vi "AngleStats_AngleMean_BiFunc.vi"(9 "B":T1, 10 "A":T1, 11 "ExtraPassedData":variant) -> (0 "Error":bool, 3 "Result":T1)   [LabVIEW 2019, in "Trajectory_Library.lvlib"]
doc: "Creates a new LINEAR SYSTEM data cluster with the specified values. \n\n\nInputs: \n - XXX -- XXX.\n\nOutputs:\n - XXX -- XXX."
uses:
  Trajectory_Library.lvlib
  <vilib>/Analysis/Matrix/Datatypes/RealMatrix.ctl
  <vilib>/Analysis/Matrix/NI_Matrix.lvlib
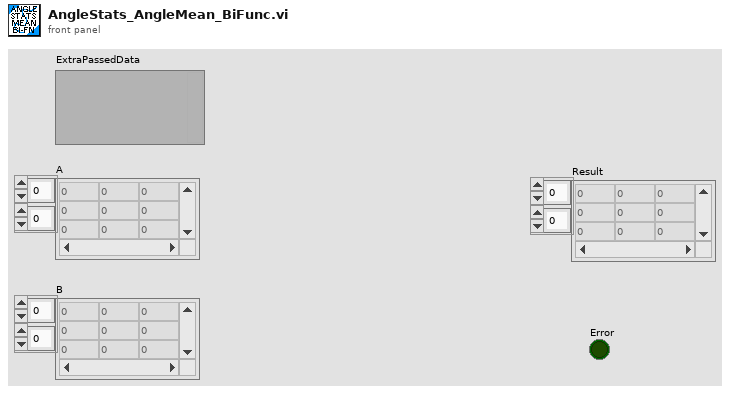
[diagram p1: front panel]
types:
  T1 = typedef "NI_Matrix.lvlib/RealMatrix.ctl" = dbl[][]
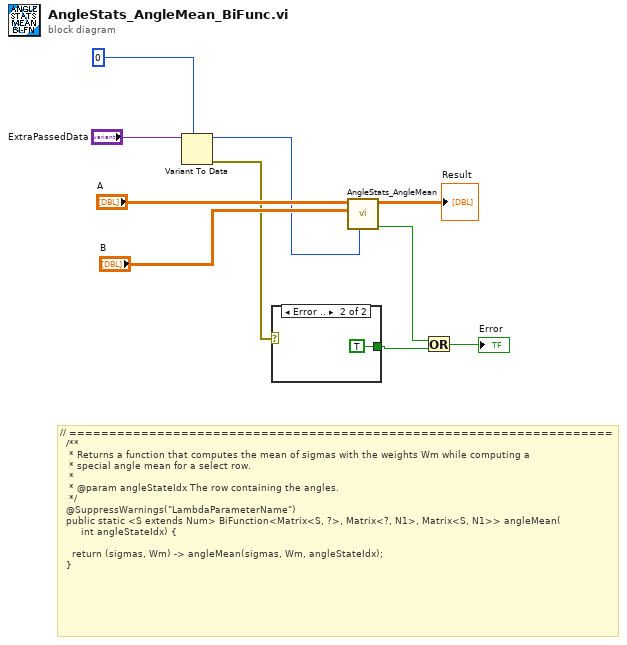
[diagram p0: block diagram]
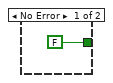
[diagram p2: hidden frame]
diagram:
  # "// ====================================================================\n  /**\n   * Returns a function that computes the mean of sigmas with the weights Wm while computing a\n   * special angle mean for a select row.\n   *\n   * @param angleStateIdx The row containing the angles.\n   */\n  @SuppressWarnings(\"LambdaParameterName\")\n  public static <S extends Num> BiFunction<Matrix<S, ?>, Matrix<?, N1>, Matrix<S, N1>> angleMean(\n      \tint angleStateIdx) {\n\n    return (sigmas, Wm) -> angleMean(sigmas, Wm, angleStateIdx);\n  }"
  n1 = Variant To Data(type=0, Variant="ExtraPassedData") -> (data=w6:i32, error out=w4:errorcluster)  [unwired: 1 in]
  n2 = case shown="Error .." w4 {
    tunnel: [FALSE TRUE] -> w2
    frame No Error {
    }
    frame Error {
    }
  }
  n3 = call "AngleStats_AngleMean.vi"("Row"=w6, "Wm"="B", "Sigmas"="A") -> ("Error"=w1:bool, "Result"=→"Result":T1)  [unwired: 7 in]
  n4 = Or(x=w1, y=w2) -> (x .or. y?=→"Error":bool)
